vi "initialWLM.vi"() -> (0 "Boolean 2":bool, 1 "Boolean":bool)   [LabVIEW 2014]
uses:
  wlmData.dll
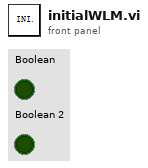
[diagram p1: front panel]
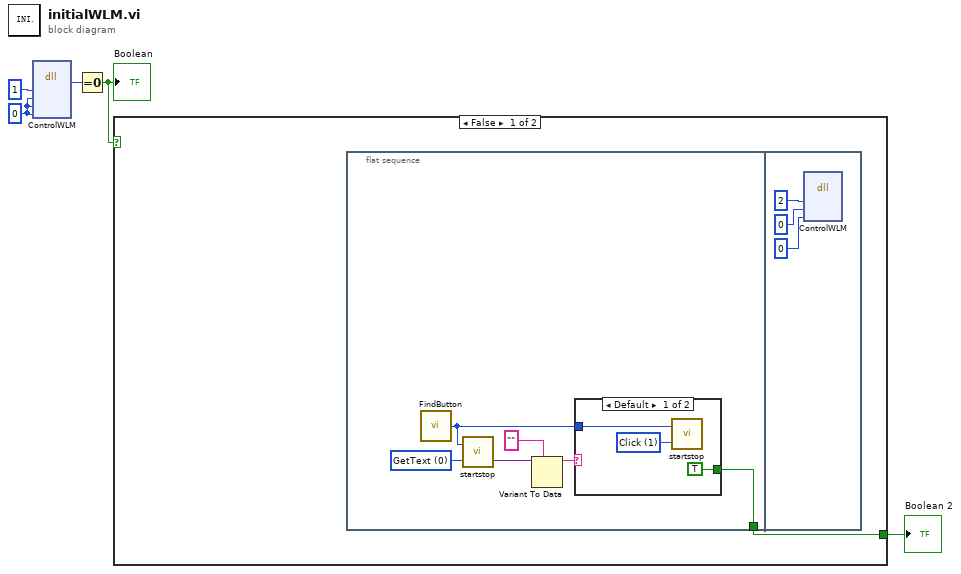
[diagram p0: block diagram]
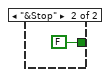
[diagram p2: hidden frame]
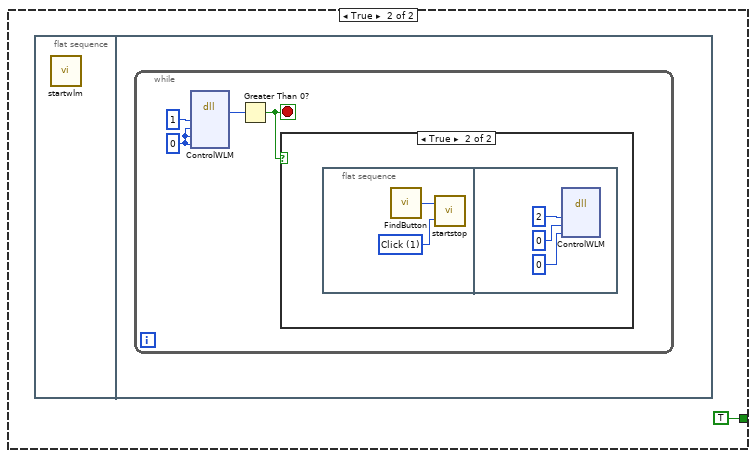
[diagram p3: hidden frame]
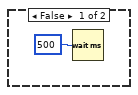
[diagram p4: hidden frame]
diagram:
  w5 = 0
  n1 = dll-call lib="wlmData.dll" fn="ControlWLM"("RFC"=1, "Mode"=w5, "p1"=w5, "p2"=w5) -> ("res"=w3:i32)  [unwired: 7 in, 2 out]
  n2 = Equal To 0?(x=w3) -> (x = 0?=w2:bool)
  "Boolean" <- w2
  n3 = case shown="False" w2 {
    tunnel: [w6 TRUE] -> w1
    frame False {
      n4 = flat-sequence {
        tunnel: [w7] -> w6
        frame #0 {
          w10 = u16 0 items=["GetText", "Click"] ("Message")
          n5 = call "FindButton.vi"() -> ("Handle"=w8:u64)
          n6 = call "startstop.vi"("Message"=w10, "Handle"=w8) -> ("Output"=w12:variant)  [unwired: 1 in]
          n7 = Variant To Data(type="", Variant=w12) -> (data=w9:string)  [unwired: 1 in, 1 out]
          n8 = case shown="Default" w9 {
            tunnel: w8 -> [w14 _]
            tunnel: [TRUE FALSE] -> w7
            frame Default {
              w15 = u16 1 items=["GetText", "Click"] ("Message")
              n9 = call "startstop.vi"("Message"=w15, "Handle"=w14) -> ()  [unwired: 1 in, 1 out]
            }
            frame "&Stop" {
            }
          }
        }
        frame #1 {
          n10 = dll-call lib="wlmData.dll" fn="ControlWLM"("action"=2, "app"=0, "ver"=0) -> ()  [unwired: 7 in, 2 out]
        }
      }
    }
    frame True {
      n11 = flat-sequence {
        frame #0 {
          n12 = call "startwlm.vi"() -> ()  [unwired: 1 in]
        }
        frame #1 {
          n13 = while {
            stop <- w21 stop-if-true
            w23 = 0
            n14 = dll-call lib="wlmData.dll" fn="ControlWLM"("RFC"=1, "Mode"=w23, "p1"=w23, "p2"=w23) -> ("res"=w22:i32)  [unwired: 7 in, 2 out]
            n15 = Greater Than 0?(x=w22) -> (x > 0?=w21:bool)
            n16 = case shown="True" w21 {
              frame False {
                n17 = Wait (ms)(milliseconds to wait=u32 500) -> ()  [unwired: 1 out]
              }
              frame True {
                n18 = flat-sequence {
                  frame #0 {
                    w26 = u16 1 items=["GetText", "Click"] ("Message")
                    n19 = call "FindButton.vi"() -> ("Handle"=w27:u64)
                    n20 = call "startstop.vi"("Message"=w26, "Handle"=w27) -> ()  [unwired: 1 in, 1 out]
                  }
                  frame #1 {
                    n21 = dll-call lib="wlmData.dll" fn="ControlWLM"("action"=2, "app"=0, "ver"=0) -> ()  [unwired: 7 in, 2 out]
                  }
                }
              }
            }
          }
        }
      }
    }
  }
  "Boolean 2" <- w1
